vi "Get Cell Indexes from Coordinates.vi"(8 "error in (no error)":errorcluster, 10 "Coordinates":cluster{"X":u32, "Y":u32}, 11 "Shape Reference":refnum<data-value>) -> (0 "error out":errorcluster, 2 "Indexes":cluster{"Row":u32, "Column":u32}, 3 "Shape Reference 2":refnum<data-value>)   [LabVIEW 2017, in "LV Image Editor Framework.lvlib" / "Grid.lvclass"]
uses:
  <vilib>/LIEF/Forms/Grid/Grid.lvclass
  <vilib>/LIEF/Forms/Shape/Shape.lvclass
  <vilib>/LIEF/Forms/Grid/Grid.lvclass/Grid.ctl
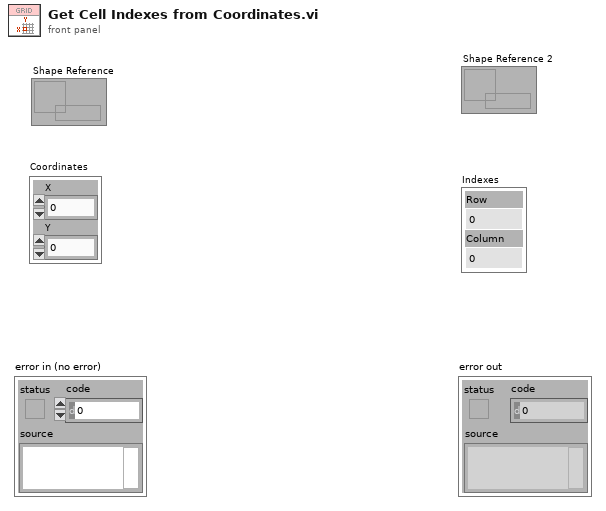
[diagram p1: front panel]
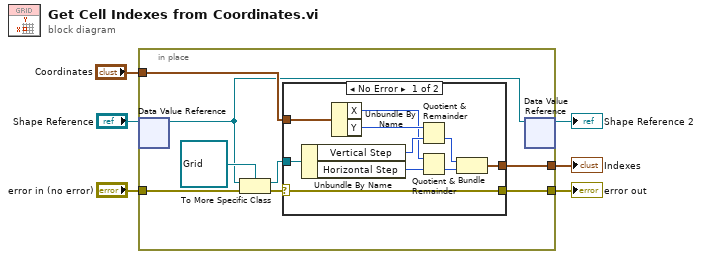
[diagram p0: block diagram]
diagram:
  n1 = in-place {
    in-place-border: "error in (no error)" -> [w9]
    in-place-border: [w14] -> w5
    in-place-border: "Coordinates" -> [w13]
    in-place-border: [w7] -> w1
    n2 = in-place-dvr #1("Shape Reference") -> (w11:refnum<class "Shape.lvclass">)  [unwired: 1 out]
    n3 = To More Specific Class(target class=refnum<class "Grid.lvclass"> refnum ("Grid in"), reference=w11, error in=w9) -> (specific class reference=w8:refnum<class "Grid.lvclass">, error out=w10:errorcluster)
    n4 = case shown="No Error" w10 {
      selector: w10 -> [w24 w25]
      tunnel: [w24 w25] -> w14
      tunnel: w8 -> [w23 _]
      tunnel: w13 -> [w22 _]
      tunnel: [w15 _] -> w7
      frame No Error {
        n5 = Unbundle By Name(w23) -> ("Vertical Step"=w21:i32, "Horizontal Step"=w20:i32)
        n6 = Unbundle By Name(w22) -> ("X"=w16:u32, "Y"=w17:u32)
        n7 = Quotient & Remainder(x=w17, y=w21) -> (floor(x/y)=w19:u32)  [unwired: 1 out]
        n8 = Quotient & Remainder(x=w16, y=w20) -> (floor(x/y)=w18:u32)  [unwired: 1 out]
        n9 = Bundle(w19, w18) -> (w15:cluster{u32, u32})  [unwired: 1 in]
      }
      frame Error {
      }
    }
    n10 = in-place-dvr #1(w11) -> (→"Shape Reference 2":refnum<data-value>)  [unwired: 1 out]
  }
  "error out" <- w5
  "Indexes" <- w1
